vi "Register for Events.vi"(8 "error in (no error)":errorcluster, 10 "This VI":refnum<vi>) -> (0 "error out":errorcluster, 1 "Stop! Event":refnum<user-event>, 2 "Event Registration Refnum":refnum<event-registration>, 3 "AbstractAutoRegistration out":refnum<class "AbstractAutoRegistration.lvclass">)   [LabVIEW 2015, in "AutoRegistration.lvlib" / "AbstractAutoRegistration.lvclass"]
uses:
  AbstractAutoRegistration.lvclass
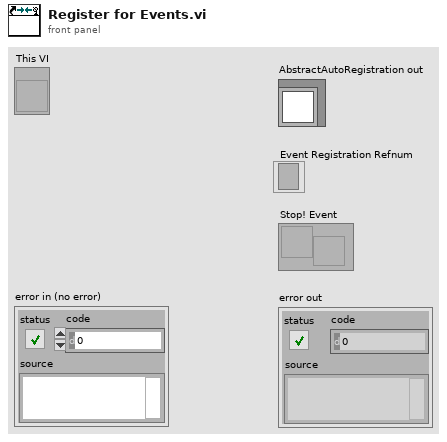
[diagram p1: front panel]
types:
  T1 = typedef "AutoRegistration.lvlib/AbstractAutoRegistration.lvclass/Registration References.ctl" = cluster{"Switching Boolean":refnum<vi>[], "Latching Boolean":refnum<vi>[], "I8":refnum<vi>[], "I16":refnum<vi>[], "I32":refnum<vi>[], "I64":refnum<vi>[], "U8":refnum<vi>[], "U16":refnum<vi>[], "U32":refnum<vi>[], "U64":refnum<vi>[], "SGL":refnum<vi>[], "DBL":refnum<vi>[], "EXT":refnum<vi>[], "FXP":refnum<vi>[], "String":refnum<vi>[], "Path":refnum<vi>[], "Timestamp":refnum<vi>[], "Other Controls":refnum<vi>[]}
  T2 = enum32{"Invalid", "Standard", "Closed", "Hidden", "Minimized", "Maximized"}
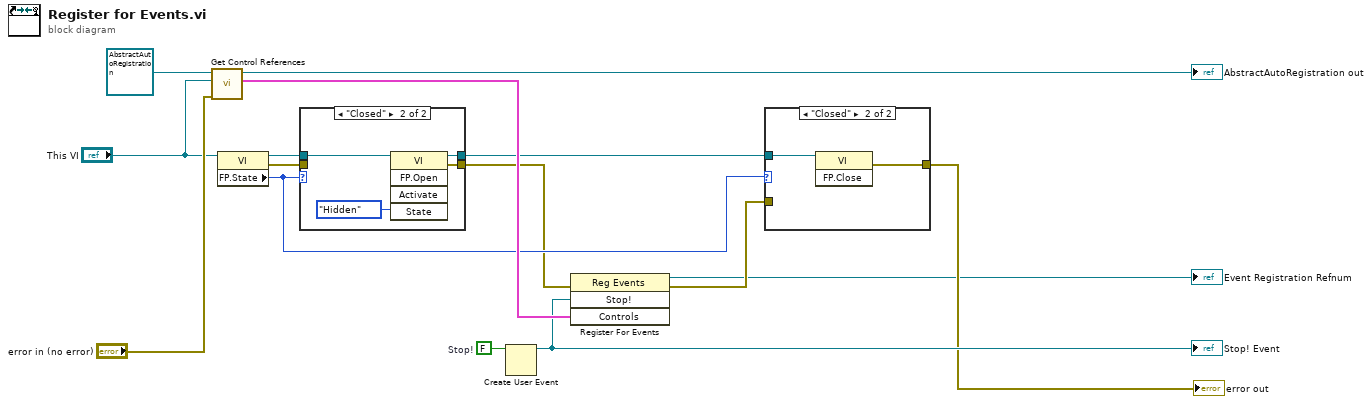
[diagram p0: block diagram]
diagram:
  w12 = FALSE  # Stop!
  n1 = call-dynamic "Get Control References.vi"("error in (no error)"="error in (no error)", "VI Refnum"="This VI", "AbstractAutoRegistration in"=refnum<class "AbstractAutoRegistration.lvclass"> refnum) -> ("Controls"=w15:T1, "AbstractAutoRegistration out"=→"AbstractAutoRegistration out":refnum<class "AbstractAutoRegistration.lvclass">)  [unwired: 6 in, 1 out]
  n2 = property on="Property Node" class="VI"(reference="This VI") -> (reference out=w10:refnum<vi>, error out=w7:errorcluster, "FP.State"=w8:T2)  [unwired: 1 in]
  n3 = case shown="\"Closed\"" w8 {
    tunnel: w10 -> [w17 w20]
    tunnel: [w16 w19] -> w6
    tunnel: [w17 w18] -> w9
    tunnel: w7 -> [w16 _]
    frame Default {
    }
    frame "Closed" {
      n4 = invoke on="Invoke Node" class="VI" method="FP.Open"(reference=w20, "State"=T2."Hidden") -> (reference out=w18:refnum<vi>, error out=w19:errorcluster)  [unwired: 3 in, 3 out]
    }
  }
  n5 = Create User Event(user event datatype=w12) -> (user event=w13:refnum<user-event>)  [unwired: 1 in, 1 out]
  "Stop! Event" <- w13
  n6 = register-events(error in=w6, w13, w15) -> (reference out=→"Event Registration Refnum":refnum<event-registration>, error out=w5:errorcluster)  [unwired: 1 in]
  n7 = case shown="\"Closed\"" w8 {
    tunnel: w9 -> [_ w23]
    tunnel: w5 -> [_ _]
    tunnel: [_ w22] -> w4
    frame Default {
    }
    frame "Closed" {
      n8 = invoke on="Invoke Node" class="VI" method="FP.Close"(reference=w23) -> (error out=w22:errorcluster)  [unwired: 2 in, 2 out]
    }
  }
  "error out" <- w4
